vi "Write Key (Variant)__ogtk.vi"(5 "float number format":string, 6 "write raw string? (F)":bool, 7 "section":string, 8 "error in (no error)":errorcluster, 9 "key-value":variant, 10 "key (optional)":string, 11 "refnum":T1) -> (0 "error out":errorcluster, 3 "refnum out":T1)   [LabVIEW 2009]
doc: "Writes a value associated with key in a specified section of the configuration data identified by refnum. If \"key\" input is not specified, the name of the variant object is used as the key.\n\nFor example a Boolean named \"Enable\" with a value of TRUE would correspond to the key-value pair:\n\nEnable=TRUE\n\nNote: Special characters in section and key names will be escape-coded. These include the following: \\00-\\1F (non-printable chars); \"[\", \"]\", and \"=\" (INI syntax elements); \\FE (\"þ\") and \\FF (\"ÿ\") (legacy bracket encoding); Additionally, the escape character, \"\\\", will be escaped as \"\\\\\"."
uses:
  <vilib>/Utility/config.llb/Config Data RefNum.ctl
  <vilib>/Utility/config.llb/Write Key (String).vi
  <vilib>/Utility/config.llb/Write Key (Path).vi
  <vilib>/Utility/config.llb/NI_LVConfig.lvlib
panel:
  in  "Ref for recursive call":refnum<vi>
  # "Write Key (Variant).vi\n\nWrites a variant key-value to INI file.\n\nPlease visit http://www.OpenG.org to learn about the\nOpen Source LabVIEW software movement.\n\nNOTICE -- YOU MUST LEAVE THIS NOTICE IN PLACE.  PER THE TERMS OF THE LICENSE BELOW, YOU MAY SUBLICENSE THIS SOFTWARE \nIN ANY WAY THAT DOES NOT CONFLICT WITH THIS LICENSE.\n\n### BSD License (http://www.opensource.org/licenses/bsd-license.php) Begin ###\n \nCopyright (c) 2002, Jean-Pierre Drolet <drolet_jp@hotmail.com>\nCopyright (c) 2002-2006, Jim Kring <jim@jimkring.com>\n\nAll rights reserved.\n\nRedistribution and use in source and binary forms, with or without modification, are permitted provided that the following conditions are met:\n\n    * Redistributions of source code must retain the above copyright notice, this list of conditions and the following disclaimer.\n    * Redistributions in binary form must reproduce the above copyright notice, this list of conditions and the following disclaimer in the \n       documentation and/or other materials provided with the distribution.\n    * Neither the name of SciWare, James Kring, Inc., nor the names of its contributors may be used to endorse or promote products derived \n       from this software without specific prior written permission.\n\nTHIS SOFTWARE IS PROVIDED BY THE COPYRIGHT HOLDERS AND CONTRIBUTORS \"AS IS\" AND ANY EXPRESS OR IMPLIED WARRANTIES, \nINCLUDING, BUT NOT LIMITED TO, THE IMPLIED WARRANTIES OF MERCHANTABILITY AND FITNESS FOR A PARTICULAR PURPOSE ARE \nDISCLAIMED. IN NO EVENT SHALL THE COPYRIGHT OWNER OR CONTRIBUTORS BE LIABLE FOR ANY DIRECT, INDIRECT, INCIDENTAL,\n SPECIAL, EXEMPLARY, OR CONSEQUENTIAL DAMAGES (INCLUDING, BUT NOT LIMITED TO, PROCUREMENT OF SUBSTITUTE GOODS OR \nSERVICES; LOSS OF USE, DATA, OR PROFITS; OR BUSINESS INTERRUPTION) HOWEVER CAUSED AND ON ANY THEORY OF LIABILITY, \nWHETHER IN CONTRACT, STRICT LIABILITY, OR TORT (INCLUDING NEGLIGENCE OR OTHERWISE) ARISING IN ANY WAY OUT OF THE USE \nOF THIS SOFTWARE, EVEN IF ADVISED OF THE POSSIBILITY OF SUCH DAMAGE.\n\n### BSD License End ###"
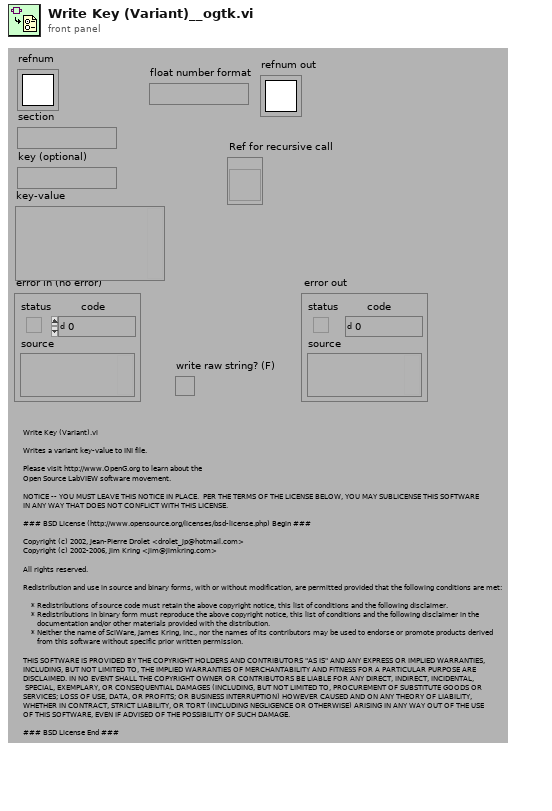
[diagram p1: front panel]
types:
  T1 = typedef "NI_LVConfig.lvlib/Config Data RefNum.ctl" = refnum<k1>
  T2 = typedef "Type Descriptor Enumeration__ogtk.ctl" = enum8{"<Null>", "I8", "I16", "I32", "I64", "U8", "U16", "U32", "U64", "SGL", "DBL", "EXT", "CSG", "CDB", "CXT", "0x0F", "0x10", "0x11", "0x12", "0x13", "0x14", "Enum U8", "Enum U16", "Enum U32", "Enum U64", "SGL PQ", "DBL PQ", "EXT PQ", "CSG PQ", "CDB PQ", "CXT PQ", "0x1F", "0x20", "Boolean", "0x22", "0x23", "0x24", "0x25", "0x26", "0x27", "0x28", "0x29", "0x2A", "0x2B", "0x2C", "0x2D", "0x2E", "0x2F", "String", "0x31", "Path", "Pict", "0x34", "0x35", "0x36", "DAQ", "0x38", "0x39", "0x3A", "0x3B", "0x3C", "0x3D", "0x3E", "0x3F", "Array", "0x41", "0x42", "0x43", "0x44", "0x45", "0x46", "0x47", "0x48", "0x49", "0x4A", "0x4B", "0x4C", "0x4D", "0x4E", "0x4F", "Cluster", "0x51", "0x52", "Variant", "Waveform", "0x55", "0x56", "0x57", "0x58", "0x59", "0x5A", "0x5B", "0x5C", "0x5D", "0x5E", "0x5F", "0x60", "0x61", "0x62", "0x63", "0x64", "0x65", "0x66", "0x67", "0x68", "0x69", "0x6A", "0x6B", "0x6C", "0x6D", "0x6E", "0x6F", "Refnum"}
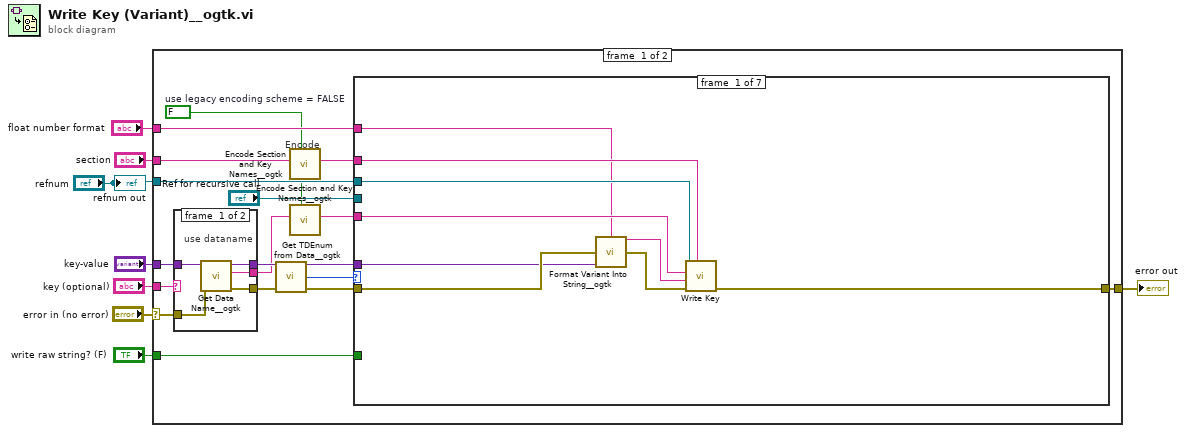
[diagram p0: block diagram]
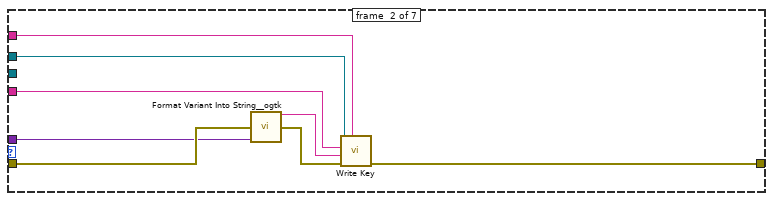
[diagram p2: hidden frame]
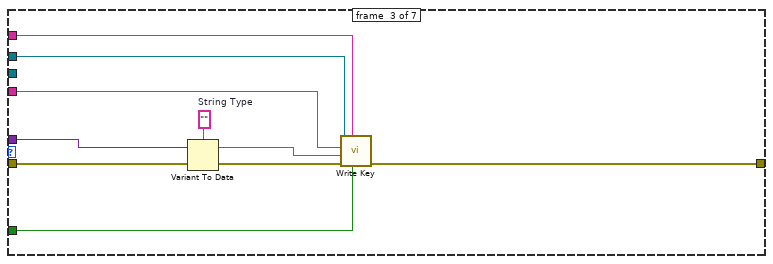
[diagram p3: hidden frame]
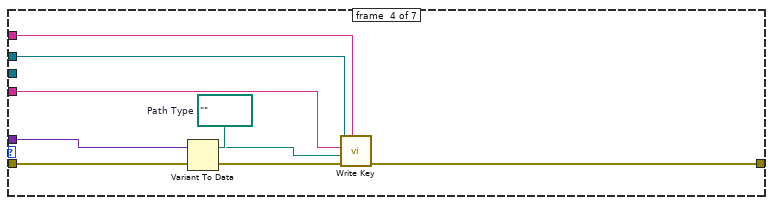
[diagram p4: hidden frame]
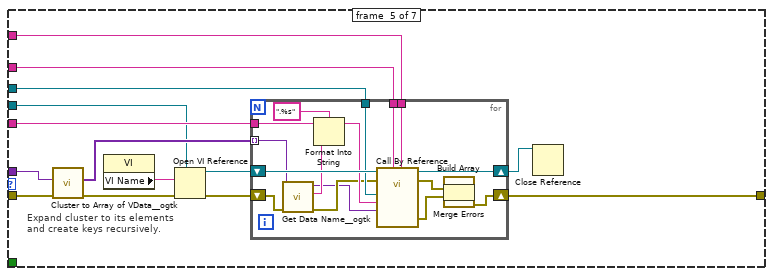
[diagram p5: hidden frame]
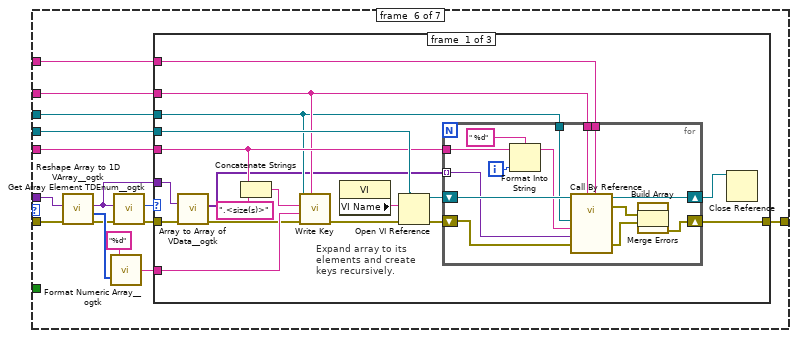
[diagram p6: hidden frame]
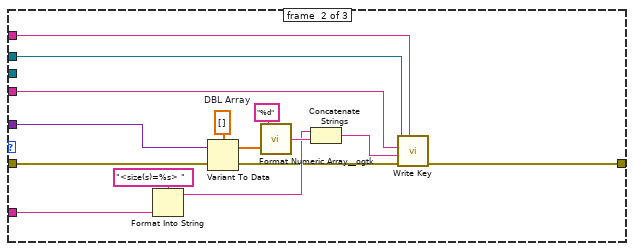
[diagram p7: hidden frame]
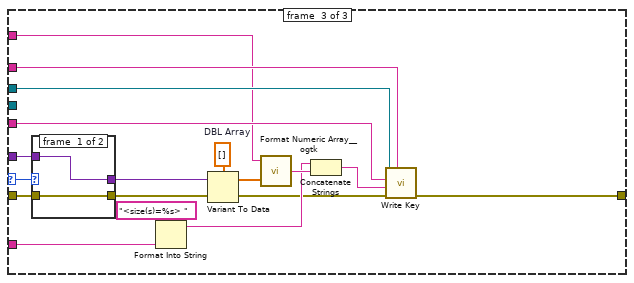
[diagram p8: hidden frame]
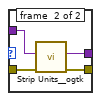
[diagram p9: hidden frame]
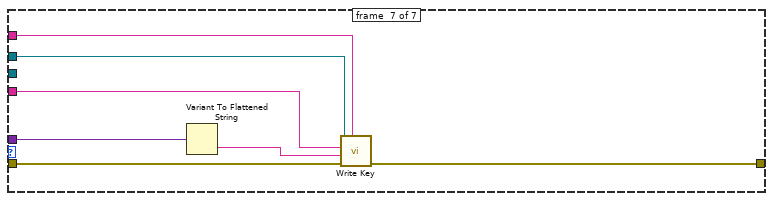
[diagram p10: hidden frame]
diagram:
  n1 = case shown="No Error" "error in (no error)" {
    selector: "error in (no error)" -> [w21 w194]
    tunnel: "refnum" -> [w24 _]
    tunnel: [w23 w194] -> w8
    tunnel: "key-value" -> [w18 _]
    tunnel: "key (optional)" -> [w22 _]
    tunnel: "section" -> [w13 _]
    tunnel: "float number format" -> [w15 _]
    tunnel: "write raw string? (F)" -> [w14 _]
    frame #0 {
      w9 = FALSE  # use legacy encoding scheme = FALSE
      # "Encode"
      n2 = case shown="\"\"" w22 {
        selector: w22 -> [_ w193]
        tunnel: [w190 w193] -> w11
        tunnel: w18 -> [w187 w191]
        tunnel: w21 -> [w189 w192]
        tunnel: [w188 w192] -> w19
        tunnel: [w186 w191] -> w17
        frame #0 {
          # "use dataname"
          n3 = call "Get Data Name__ogtk.vi"("error in (no error)"=w189, "Data"=w187) -> ("error out"=w188:errorcluster, "Data Name"=w190:string, "Data dup"=w186:variant)  [unwired: 7 in]
        }
        frame #1 {
          # "use optional\nkey"
        }
      }
      n4 = call "Get TDEnum from Data__ogtk.vi"("Data"=w17) -> ("Type Descriptor Enumeration"=w20:T2)  [unwired: 4 in]
      n5 = call "Encode Section and Key Names__ogtk.vi"("use legacy encoding scheme? (FALSE)"=w9, "string"=w13) -> ("encoded string"=w12:string)  [unwired: 9 in]
      n6 = call "Encode Section and Key Names__ogtk.vi"("use legacy encoding scheme? (FALSE)"=w9, "string"=w11) -> ("encoded string"=w10:string)  [unwired: 9 in]
      n7 = case shown="\"String\", \"DAQ\"" w20 {
        tunnel: w17 -> [w28 w36 w49 w58 w67 w104 w181]
        tunnel: w24 -> [w33 w41 w48 w57 w71 w98 w185]
        tunnel: [w32 w40 w46 w55 w69 w106 w184] -> w23
        tunnel: w19 -> [w29 w37 w45 w54 w66 w103 w180]
        tunnel: w10 -> [w31 w39 w44 w53 w63 w97 w183]
        tunnel: w12 -> [w30 w38 w43 w52 w70 w99 w182]
        tunnel: "Ref for recursive call" -> [_ _ _ _ w62 w105 _]
        tunnel: w15 -> [w27 _ _ _ w61 w92 _]
        tunnel: w14 -> [_ _ w42 _ _ _ _]
        frame #0 {
          n8 = call "Format Variant Into String__ogtk.vi"("Format String"=w27, "error in (no error)"=w29, "Variant"=w28) -> ("Output String"=w25:string, "error out"=w26:errorcluster)  [unwired: 11 in]
          n9 = call-poly <vilib>:"Write Key.vi"("section"=w30, "error in (no error)"=w26, "value"=w25, "key"=w31, "refnum"=w33) -> ("error out"=w32:errorcluster)  [unwired: 4 in, 2 out]
        }
        frame #1 {
          n10 = call "Format Variant Into String__ogtk.vi"("error in (no error)"=w37, "Variant"=w36) -> ("Output String"=w34:string, "error out"=w35:errorcluster)  [unwired: 12 in]
          n11 = call-poly <vilib>:"Write Key.vi"("section"=w38, "error in (no error)"=w35, "value"=w34, "key"=w39, "refnum"=w41) -> ("error out"=w40:errorcluster)  [unwired: 4 in, 2 out]
        }
        frame #2 {
          w51 = ""  # String Type
          n12 = Variant To Data(error in=w45, Variant=w49, type=w51) -> (error out=w47:errorcluster, data=w50:string)
          n13 = call-poly <vilib>:"Write Key.vi"("write raw string? (F)"=w42, "section"=w43, "error in (no error)"=w47, "value"=w50, "key"=w44, "refnum"=w48) -> ("error out"=w46:errorcluster)  [unwired: 3 in, 2 out]
        }
        frame #3 {
          w60 = path ""  # Path Type
          n14 = Variant To Data(error in=w54, Variant=w58, type=w60) -> (error out=w56:errorcluster, data=w59:path)
          n15 = call-poly <vilib>:"Write Key.vi"("section"=w52, "error in (no error)"=w56, "value"=w59, "key"=w53, "refnum"=w57) -> ("error out"=w55:errorcluster)  [unwired: 4 in, 2 out]
        }
        frame #4 {
          # "Expand cluster to its elements\nand create keys recursively."
          n16 = call "Cluster to Array of VData__ogtk.vi"("error in (no error)"=w66, "Cluster"=w67) -> ("error out"=w64:errorcluster, "Array of VData"=w65:variant[])  [unwired: 8 in]
          n17 = property class="VI"() -> ("VI Name"=w68:string)  [unwired: 2 in, 2 out]
          n18 = Open VI Reference(type specifier VI Refnum (for type only)=w62, vi path=w68, error in (no error)=w64) -> (vi reference=w74:refnum<vi>, error out=w72:errorcluster)  [unwired: 3 in]
          n19 = for {
            shift-right: [w90] -> w73
            shift-left: w74 -> [w91]
            shift-right: [w85] -> w69
            shift-left: w72 -> [w80]
            tunnel: w65 -> [w78] mode=indexing
            tunnel: w70 -> [w89]
            tunnel: w71 -> [w88]
            tunnel: w63 -> [w84]
            tunnel: w61 -> [w76]
            n20 = call "Get Data Name__ogtk.vi"("error in (no error)"=w80, "Data"=w78) -> ("error out"=w79:errorcluster, "Data Name"=w83:string, "Data dup"=w77:variant)  [unwired: 7 in]
            n21 = Format Into String(format string=".%s" ("Format String"), initial string=w84, w83) -> (resulting string=w82:string)  [unwired: 1 in, 1 out]
            n22 = call-by-ref "?"(reference=w91, error in=w79, "format string"=w76, "section"=w89, "key-value"=w77, "key (optional)"=w82, "refnum"=w88) -> (reference out=w90:refnum<vi>, error out=w86:errorcluster, "error out"=w87:errorcluster)  [unwired: 5 in, 1 out]
            n23 = Build Array(w86, w87) -> (w75:errorcluster[])
            n24 = call <vilib>:"Merge Errors.vi"("error array in"=w75) -> ("error out"=w85:errorcluster)  [unwired: 6 in]
          }
          n25 = Close Reference(reference=w73) -> ()  [unwired: 1 in, 1 out]
        }
        frame #5 {
          n26 = call "Reshape Array to 1D VArray__ogtk.vi"("error in (no error)"=w103, "MultiD Array"=w104) -> ("error out"=w93:errorcluster, "Size(s)"=w101:u32[], "1D VArray"=w94:variant)  [unwired: 7 in]
          n27 = call "Format Numeric Array__ogtk.vi"("Array"=w101, "format string"="%d") -> ("Formatted on a line"=w95:string)
          n28 = call "Get Array Element TDEnum__ogtk.vi"("error in (no error)"=w93, "Array"=w94) -> ("error out"=w96:errorcluster, "Element Type"=w100:T2)  [unwired: 8 in]
          n29 = case shown="\"I8\"..\"I32\", \"U8\"..\"U32\"" w100 {
            selector: w100 -> [_ _ w160]
            tunnel: w98 -> [w114 w143 w163]
            tunnel: w99 -> [w115 w144 w164]
            tunnel: [w121 w141 w161] -> w106
            tunnel: w97 -> [w118 w142 w162]
            tunnel: w105 -> [w119 _ _]
            tunnel: w96 -> [w111 w145 w159]
            tunnel: w95 -> [w112 w146 w165]
            tunnel: w94 -> [w109 w140 w157]
            tunnel: w92 -> [w107 _ w155]
            frame #0 {
              # "Expand array to its\nelements and create\nkeys recursively."
              n30 = call "Array to Array of VData__ogtk.vi"("error in (no error)"=w111, "MultiD Array"=w109) -> ("error out"=w110:errorcluster, "1D Array of Variants"=w108:variant[])  [unwired: 8 in]
              n31 = Concatenate Strings(w118, ".<size(s)>" ("Substring")) -> (w113:string)
              n32 = call-poly <vilib>:"Write Key.vi"("section"=w115, "error in (no error)"=w110, "value"=w112, "key"=w113, "refnum"=w114) -> ("error out"=w117:errorcluster)  [unwired: 4 in, 2 out]
              n33 = property class="VI"() -> ("VI Name"=w120:string)  [unwired: 2 in, 2 out]
              n34 = Open VI Reference(type specifier VI Refnum (for type only)=w119, vi path=w120, error in (no error)=w117) -> (vi reference=w124:refnum<vi>, error out=w122:errorcluster)  [unwired: 3 in]
              n35 = for {
                shift-right: [w138] -> w123
                shift-left: w124 -> [w139]
                shift-right: [w133] -> w121
                shift-left: w122 -> [w128]
                tunnel: w108 -> [w129] mode=indexing
                tunnel: w115 -> [w137]
                tunnel: w114 -> [w136]
                tunnel: w118 -> [w132]
                tunnel: w107 -> [w126]
                i -> [w127]
                n36 = Format Into String(format string=" %d" ("Format String"), initial string=w132, w127) -> (resulting string=w131:string)  [unwired: 1 in, 1 out]
                n37 = call-by-ref "?"(reference=w139, "format string"=w126, "section"=w137, "error in (no error)"=w128, "key-value"=w129, "key (optional)"=w131, "refnum"=w136) -> (reference out=w138:refnum<vi>, error out=w134:errorcluster, "error out"=w135:errorcluster)  [unwired: 5 in, 1 out]
                n38 = Build Array(w134, w135) -> (w125:errorcluster[])
                n39 = call <vilib>:"Merge Errors.vi"("error array in"=w125) -> ("error out"=w133:errorcluster)  [unwired: 6 in]
              }
              n40 = Close Reference(reference=w123) -> ()  [unwired: 1 in, 1 out]
            }
            frame #1 {
              w154 = dbl[] []  # DBL Array
              n41 = Format Into String(format string="<size(s)=%s> " ("Format String"), w146) -> (resulting string=w149:string)  [unwired: 2 in, 1 out]
              n42 = Variant To Data(error in=w145, Variant=w140, type=w154) -> (error out=w148:errorcluster, data=w153:dbl[])
              n43 = call "Format Numeric Array__ogtk.vi"("Array"=w153, "format string"="%d") -> ("Formatted on a line"=w152:string)
              n44 = Concatenate Strings(w149, w152) -> (w147:string)
              n45 = call-poly <vilib>:"Write Key.vi"("section"=w144, "error in (no error)"=w148, "value"=w147, "key"=w142, "refnum"=w143) -> ("error out"=w141:errorcluster)  [unwired: 4 in, 2 out]
            }
            frame #2 {
              w172 = dbl[] []  # DBL Array
              n46 = case shown="\"SGL PQ\"..\"EXT PQ\"" w160 {
                tunnel: w159 -> [w174 w178]
                tunnel: [w174 w177] -> w158
                tunnel: w157 -> [w173 w176]
                tunnel: [w173 w175] -> w156
                frame #0 {
                }
                frame #1 {
                  n47 = call "Strip Units__ogtk.vi"("error in (no error)"=w178, "Number or 1D array with units"=w176) -> ("error out"=w177:errorcluster, "Pure Number(s) (base units)"=w175:variant)  [unwired: 8 in]
                }
              }
              n48 = Format Into String(format string="<size(s)=%s> " ("Format String"), w165) -> (resulting string=w168:string)  [unwired: 2 in, 1 out]
              n49 = Variant To Data(error in=w158, Variant=w156, type=w172) -> (error out=w167:errorcluster, data=w171:dbl[])
              n50 = call "Format Numeric Array__ogtk.vi"("Array"=w171, "format string"=w155) -> ("Formatted on a line"=w170:string)
              n51 = Concatenate Strings(w168, w170) -> (w166:string)
              n52 = call-poly <vilib>:"Write Key.vi"("section"=w164, "error in (no error)"=w167, "value"=w166, "key"=w162, "refnum"=w163) -> ("error out"=w161:errorcluster)  [unwired: 4 in, 2 out]
            }
          }
        }
        frame #6 {
          n53 = Variant To Flattened String(Variant=w181) -> (data string=w179:string)  [unwired: 1 out]
          n54 = call-poly <vilib>:"Write Key.vi"("section"=w182, "error in (no error)"=w180, "value"=w179, "key"=w183, "refnum"=w185) -> ("error out"=w184:errorcluster)  [unwired: 4 in, 2 out]
        }
      }
    }
    frame #1 {
    }
  }
  "error out" <- w8
  "refnum out" <- "refnum"
